vi "AFG_Init.vi"(1 "amplitude (1)":dbl=1.0, 2 "resource name":refnum<k15>="USB0::0x0699::0x0340::C012041::INSTR", 3 "frequency (1000000)":dbl=100.0) -> (0 "instrument handle out":refnum<k15>)   [LabVIEW 2010]
panel:
  out "error out":errorcluster {"code" format="%.0x"}
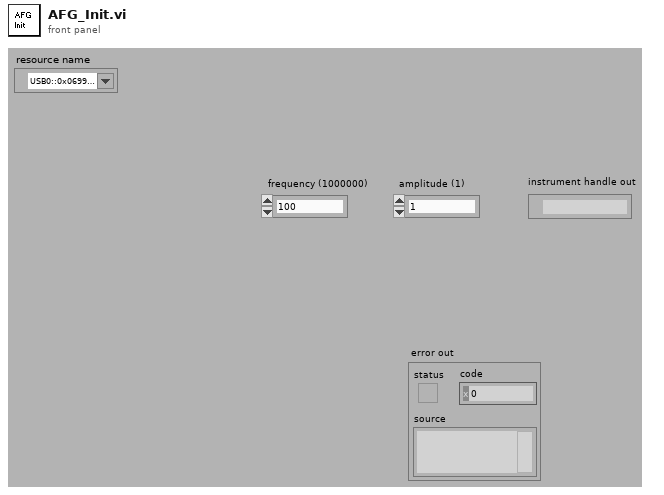
[diagram p1: front panel]
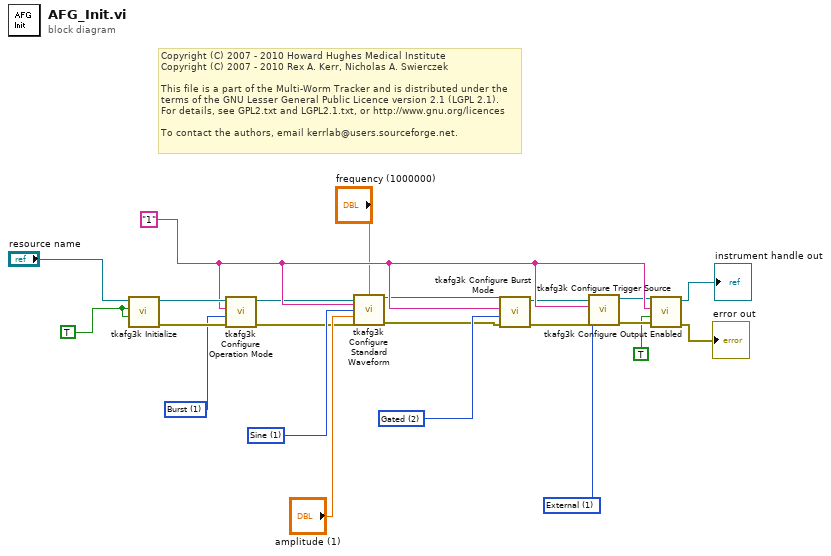
[diagram p0: block diagram]
diagram:
  w15 = 2 items=["Triggered"=1, "Gated"=2] ("Burst Mode (Triggered)")
  w16 = 1 items=["Continuous"=0, "Modulation"=1001, "Sweep"=1002, "Burst"=1] ("operation mode (Continuous)")
  w13 = 1 items=["Sine"=1, "Square"=2, "Pulse"=1002, "Ramp"=1001, "Noise"=1003, "DC"=6, "Sin(x)/x"=1004, "Gaussian"=1005, "Lorentz"=1006, "Exponential Rise"=1007, "Exponential Decay"=1008, "Haversine"=1009] ("waveform (Sine)")
  w8 = 1 items=["External"=1, "Internal"=3] ("trigger source (External)")
  w17 = "1"
  w19 = TRUE ("id query (Yes)")
  # "Copyright (C) 2007 - 2010 Howard Hughes Medical Institute\nCopyright (C) 2007 - 2010 Rex A. Kerr, Nicholas A. Swierczek\n \nThis file is a part of the Multi-Worm Tracker and is distributed under the\nterms of the GNU Lesser General Public Licence version 2.1 (LGPL 2.1).\nFor details, see GPL2.txt and LGPL2.1.txt, or http://www.gnu.org/licences\n \nTo contact the authors, email kerrlab@users.sourceforge.net."
  n1 = call <instrlib>:"tkafg3k Initialize.vi"("reset device (Yes)"=w19, "id query (Yes)"=w19, "resource name"="resource name") -> ("error out"=w20:errorcluster, "instrument handle out"=w21:refnum<k15>)  [unwired: 7 in]
  n2 = call <instrlib>:"tkafg3k Configure Operation Mode.vi"("error in (no error)"=w20, "operation mode (Continuous)"=w16, "channel name (\"1\")"=w17, "instrument handle"=w21) -> ("error out"=w2:errorcluster, "instrument handle out"=w3:refnum<k15>)  [unwired: 6 in]
  n3 = call <instrlib>:"tkafg3k Configure Standard Waveform.vi"("instrument handle"=w3, "frequency (1000000)"="frequency (1000000)", "channel name (\"1\")"=w17, "waveform (Sine)"=w13, "amplitude (1)"="amplitude (1)", "error in (no error)"=w2) -> ("instrument handle out"=w11:refnum<k15>, "error out"=w10:errorcluster)  [unwired: 8 in]
  n4 = call <instrlib>:"tkafg3k Configure Burst Mode.vi"("error in (no error)"=w10, "Burst Mode (Triggered)"=w15, "Channel Name (\"1\")"=w17, "instrument handle"=w11) -> ("error out"=w7:errorcluster, "instrument handle out"=w9:refnum<k15>)  [unwired: 6 in]
  n5 = call <instrlib>:"tkafg3k Configure Trigger Source.vi"("error in (no error)"=w7, "trigger source (External)"=w8, "channel name (\"1\")"=w17, "instrument handle"=w9) -> ("error out"=w6:errorcluster, "instrument handle out"=w5:refnum<k15>)  [unwired: 6 in]
  n6 = call <instrlib>:"tkafg3k Configure Output Enabled.vi"("error in (no error)"=w6, "channel enabled (True)"=TRUE, "channel name (\"1\")"=w17, "instrument handle"=w5) -> ("error out"=→"error out":errorcluster, "instrument handle out"=→"instrument handle out":refnum<k15>)  [unwired: 6 in]
